vi "Click Event.vi"(8 "error in (no error)":errorcluster, 9 "Event Data":variant, 11 "Button in":refnum<class "Button.lvclass">) -> (0 "error out":errorcluster, 2 "Value Changed ?":bool, 3 "Button out":refnum<class "Button.lvclass">)   [LabVIEW 2012, in "Button.lvclass"]
doc: "The button method that is actually called when the a button is clicked/latched or unlatched. This is where one would hook an custom actions by overiding this method."
uses:
  Button.lvclass
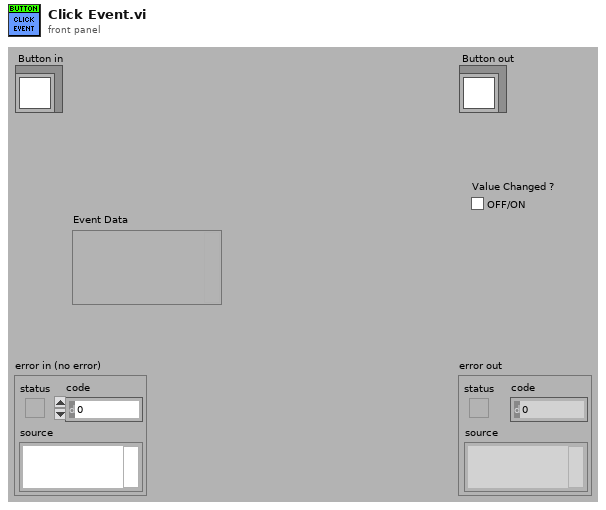
[diagram p1: front panel]
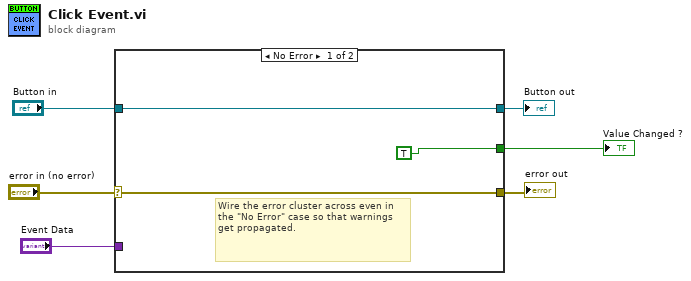
[diagram p0: block diagram]
diagram:
  n1 = case shown="No Error" "error in (no error)" {
    selector: "error in (no error)" -> [w8 w11]
    tunnel: [w8 w11] -> w5
    tunnel: [w9 w10] -> w3
    tunnel: "Button in" -> [w9 w10]
    tunnel: "Event Data" -> [_ _]
    tunnel: [TRUE _] -> w1
    frame No Error {
      # "Wire the error cluster across even in the \"No Error\" case so that warnings get propagated."
    }
    frame Error {
    }
  }
  "error out" <- w5
  "Button out" <- w3
  "Value Changed ?" <- w1
